vi "destoryChildEvents.vi"(8 "error in (no error)":errorcluster, 11 "CommandEvents in":refnum<class "CommandEvents.lvclass">) -> (0 "error out":errorcluster, 3 "CommandEvents out":refnum<class "CommandEvents.lvclass">)   [LabVIEW 2009, in "Tools.lvlib" / "Interpreters.lvlib" / "CommandEvents.lvclass"]
uses:
  CommandEvents.lvclass
  CommandEvents.lvclass/CommandEvents.ctl
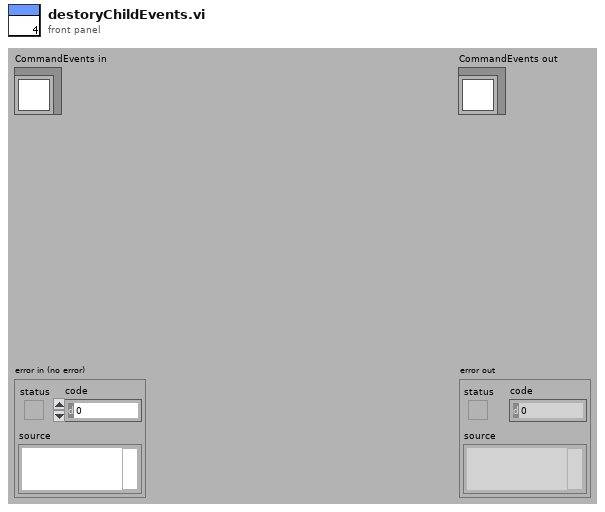
[diagram p1: front panel]
types:
  T1 = cluster{"newCommand":refnum<user-event>, "textUpdate":refnum<user-event>}
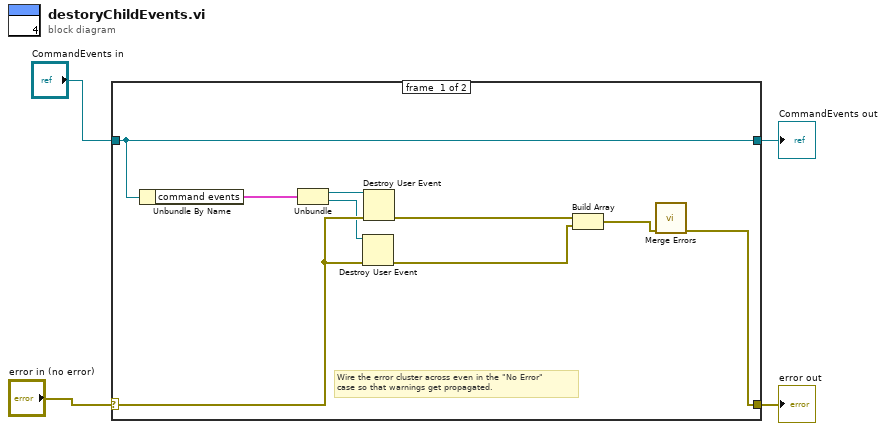
[diagram p0: block diagram]
diagram:
  n1 = case shown="No Error" "error in (no error)" {
    selector: "error in (no error)" -> [w11 w15]
    tunnel: [w7 w15] -> w3
    tunnel: [w6 w14] -> w1
    tunnel: "CommandEvents in" -> [w6 w14]
    frame #0 {
      # "Wire the error cluster across even in the \"No Error\"\ncase so that warnings get propagated."
      n2 = Unbundle By Name(w6) -> ("command events"=w5:T1)
      n3 = Unbundle(w5) -> ("newCommand"=w12:refnum<user-event>, "textUpdate"=w10:refnum<user-event>)
      n4 = Destroy User Event(user event=w10, error in=w11) -> (error out=w9:errorcluster)
      n5 = Destroy User Event(user event=w12, error in=w11) -> (error out=w13:errorcluster)
      n6 = Build Array(w13, w9) -> (w8:errorcluster[])
      n7 = call <vilib>:"Merge Errors.vi"("error array in"=w8) -> ("error out"=w7:errorcluster)  [unwired: 6 in]
    }
    frame #1 {
    }
  }
  "error out" <- w3
  "CommandEvents out" <- w1
